vi "GenericDataCfg.vi"(7 "Write?":bool, 8 "error in":errorcluster, 11 "CfgFileIn":T1) -> (0 "error out":errorcluster, 3 "CfgFileOut":T1)   [LabVIEW 2012]
uses:
  <vilib>/Utility/config.llb/NI_LVConfig.lvlib
  <vilib>/Utility/config.llb/Write Key (String).vi
  <vilib>/Utility/config.llb/Read Key (Boolean).vi
  <vilib>/Utility/config.llb/Config Data RefNum.ctl
panel:
  in  "Ctl Refnum":refnum<vi>
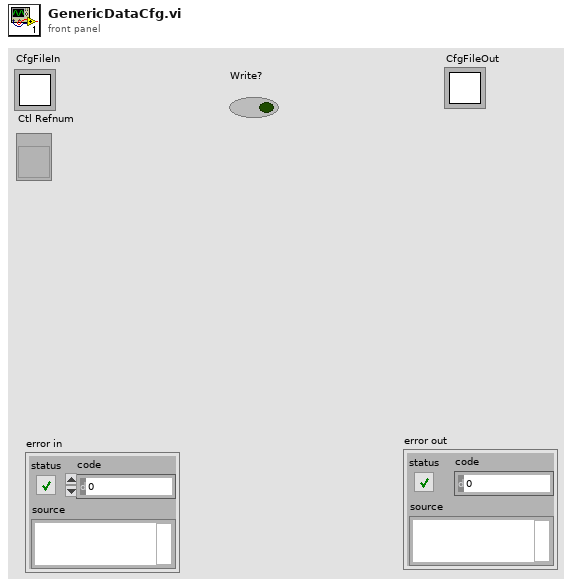
[diagram p1: front panel]
types:
  T1 = typedef "NI_LVConfig.lvlib/Config Data RefNum.ctl" = refnum<k1>
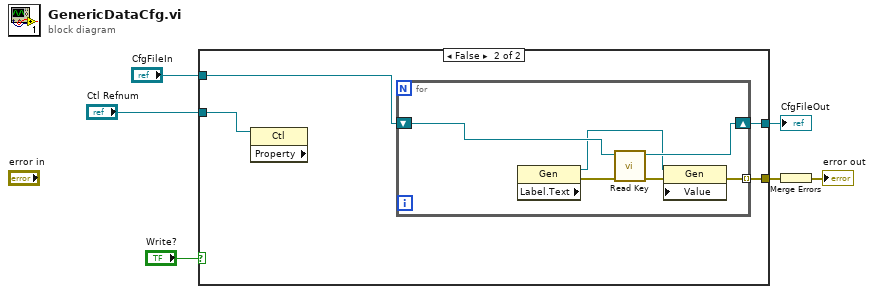
[diagram p0: block diagram]
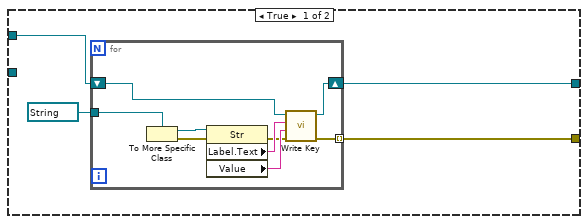
[diagram p2: hidden frame]
diagram:
  n1 = case shown="False" "Write?" {
    tunnel: "CfgFileIn" -> [w9 w23]
    tunnel: [w8 w22] -> w5
    tunnel: [w7 w21] -> w4
    tunnel: "Ctl Refnum" -> [_ w20]
    frame True {
      n2 = for {
        tunnel: refnum<vi> refnum ("Str Refnum") -> [w19]
        shift-right: [w13] -> w8
        shift-left: w9 -> [w16]
        tunnel: [w11] -> w7 mode=indexing
        n3 = To More Specific Class(target class=w19) -> (specific class reference=w18:refnum<vi>, error out=w17:errorcluster)  [unwired: 2 in]
        n4 = property class="Str"(reference=w18, error in=w17) -> (error out=w12:errorcluster, "Label.Text"=w15:string, "Value"=w14:string)  [unwired: 1 out]
        n5 = call-poly <vilib>:"Write Key.vi"("error in (no error)"=w12, "value"=w14, "key"=w15, "refnum"=w16) -> ("error out"=w11:errorcluster, "refnum out"=w13:T1)  [unwired: 5 in, 1 out]
      }
    }
    frame False {
      n6 = property class="Ctl" props=[](reference=w20) -> ()  [unwired: 1 in, 3 out]
      n7 = for {
        shift-right: [w28] -> w22
        shift-left: w23 -> [w29]
        tunnel: [w24] -> w21 mode=indexing
        n8 = property class="Gen" props=["Label", "Text"]() -> (reference out=w26:refnum<vi>, error out=w27:errorcluster)  [unwired: 2 in, 1 out]
        n9 = call-poly <vilib>:"Read Key.vi"("error in (no error)"=w27, "refnum"=w29) -> ("error out"=w25:errorcluster, "refnum out"=w28:T1)  [unwired: 6 in, 2 out]
        n10 = property class="Gen" props=["Value"](reference=w26, error in=w25) -> (error out=w24:errorcluster)  [unwired: 1 in, 1 out]
      }
    }
  }
  "CfgFileOut" <- w5
  n11 = Merge Errors(w4) -> (→"error out":errorcluster)
